vi "Data Acquisition.vi"() -> ()   [LabVIEW 2019]
uses:
  <vilib>/vision/Avi.llb/IMAQ AVI2 Refnum.ctl
  <vilib>/vision/Image Controls.llb/IMAQ Image.ctl
  <vilib>/Instr/_visa.llb/VISA Configure Serial Port (Instr).vi
panel:
  out "slowdata2":refnum<queue>
  out "slow frame":T1
  out "String":string="file:///C:\\Users\\ThymeLab\\Desktop\\omr_movies\\vdark50_vlight200_Rev.avi"
  in  "stop 2":bool
  in  "VLC Reference":refnum<k7>
  out "COMport":refnum<visa-resource-name>="COM4"
  out "hsframe":T1
  out "AVI Refnum":T2
  out "time log":refnum<file>
  out "slowdata":refnum<queue>
  out "integral1":refnum<queue>
  out "centroids1":refnum<queue>
  out "slowdisplay":refnum<queue>
  out "threshDisplay1":refnum<queue>
  in  "Tab Control":enum32{"Main View", "Files to load/save"}(tab)=enum."Files to load/save"
  out "Image":T1(plugin-control)
  in  "Ring":u16(ring) items=["Raw", "Diff Threshold", "Integrated Motion"]
  in  "stop":bool
  out "Buffers":i32(slide) scale=0.0..100.0
  out "Intensity Graph":u32[][](graph)
  out "movieindex":dbl
  in  "High Speed Movie Path":path=path "C:/Users/ThymeLab/Desktop/Box12/hsmovie"
  in  "ROI Refernce Image 1":path=path "C:/Users/ThymeLab/Desktop/Box12/Box12.png"
  in  "Load Experimental Parameters":path=path "C:/Users/ThymeLab/Desktop/Box12/fulltestrun_final_01_27_2020"
  in  "Load ROI Data":path=path "C:/Users/ThymeLab/Desktop/Box12/rois"
  in  "Log File Base Name":path=path "C:/Users/ThymeLab/Desktop/Box12/testlog"
  in  "diff threshold":dbl=3.0
  out "modhspath":path=path "C:/Users/ThymeLab/Desktop/Box1/hsmovieSun, Jun 14, 2020"
  in  "Teensy COM":refnum<visa-resource-name>="COM3"
  out "doQueue1":refnum<queue>
  out "hsdata":refnum<queue>
  in  "Folder containing stimulaton movies":path
  in  "Movie to Play":dbl
  in  "Pause":bool
  out "motion log":refnum<file>
  out "centroid log":refnum<file>
  out "ROIs":T3={[0, 0, 1088, 660], [{"Contour Type"=0, "ROI Type"=12, [32, 2, 115, 83, 90000]}, {"Contour Type"=0, "ROI Type"=12, [32, 83, 115, 164, 90000]}, {"Contour Type"=0, "ROI Type"=12, [32, 165, 115, 246, 90000]}, {"Contour Type"=0, "ROI Type"=12, [32, 246, 115, 327, 90000]}, {"Contour Type"=0, "ROI Type"=12, [32, 328, 116, 408, 90000]}, {"Contour Type"=0, "ROI Type"=12, [33, 409, 116, 490, 90000]}, {"Contour Type"=0, "ROI Type"=12, [33, 490, 116, 571, 90000]}, {"Contour Type"=0, "ROI Type"=12, [33, 572, 116, 653, 90000]}, {"Contour Type"=0, "ROI Type"=12, [116, 2, 199, 83, 90000]}, {"Contour Type"=0, "ROI Type"=12, [116, 83, 199, 164, 90000]}, {"Contour Type"=0, "ROI Type"=12, [116, 165, 199, 246, 90000]}, {"Contour Type"=0, "ROI Type"=12, [116, 246, 199, 327, 90000]}, {"Contour Type"=0, "ROI Type"=12, [116, 328, 199, 408, 90000]}, {"Contour Type"=0, "ROI Type"=12, [116, 409, 199, 490, 90000]}, {"Contour Type"=0, "ROI Type"=12, [116, 490, 199, 571, 90000]}, {"Contour Type"=0, "ROI Type"=12, [117, 572, 200, 653, 90000]}, {"Contour Type"=0, "ROI Type"=12, [199, 2, 282, 83, 90000]}, {"Contour Type"=0, "ROI Type"=12, [199, 83, 282, 164, 90000]}, {"Contour Type"=0, "ROI Type"=12, [200, 165, 283, 246, 90000]}, {"Contour Type"=0, "ROI Type"=12, [200, 246, 283, 327, 90000]}, {"Contour Type"=0, "ROI Type"=12, [200, 328, 283, 408, 90000]}, {"Contour Type"=0, "ROI Type"=12, [200, 409, 283, 490, 90000]}, {"Contour Type"=0, "ROI Type"=12, [200, 490, 283, 571, 90000]}, {"Contour Type"=0, "ROI Type"=12, [200, 572, 283, 653, 90000]}, {"Contour Type"=0, "ROI Type"=12, [283, 2, 366, 83, 90000]}, {"Contour Type"=0, "ROI Type"=12, [283, 83, 366, 164, 90000]}, {"Contour Type"=0, "ROI Type"=12, [283, 165, 366, 246, 90000]}, {"Contour Type"=0, "ROI Type"=12, [283, 246, 366, 327, 90000]}, {"Contour Type"=0, "ROI Type"=12, [284, 328, 366, 408, 90000]}, {"Contour Type"=0, "ROI Type"=12, [284, 409, 367, 490, 90000]}, {"Contour Type"=0, "ROI Type"=12, [284, 490, 367, 571, 90000]}, {"Contour Type"=0, "ROI Type"=12, [284, 572, 367, 653, 90000]}, {"Contour Type"=0, "ROI Type"=12, [367, 2, 450, 83, 90000]}, {"Contour Type"=0, "ROI Type"=12, [367, 83, 450, 164, 90000]}, {"Contour Type"=0, "ROI Type"=12, [367, 165, 450, 246, 90000]}, {"Contour Type"=0, "ROI Type"=12, [367, 246, 450, 327, 90000]}, {"Contour Type"=0, "ROI Type"=12, [367, 328, 450, 408, 90000]}, {"Contour Type"=0, "ROI Type"=12, [367, 409, 450, 490, 90000]}, {"Contour Type"=0, "ROI Type"=12, [367, 490, 450, 571, 90000]}, {"Contour Type"=0, "ROI Type"=12, [368, 572, 451, 653, 90000]}, {"Contour Type"=0, "ROI Type"=12, [450, 2, 533, 83, 90000]}, {"Contour Type"=0, "ROI Type"=12, [450, 83, 533, 164, 90000]}, {"Contour Type"=0, "ROI Type"=12, [451, 165, 534, 246, 90000]}, {"Contour Type"=0, "ROI Type"=12, [451, 246, 534, 327, 90000]}, {"Contour Type"=0, "ROI Type"=12, [451, 328, 534, 408, 90000]}, {"Contour Type"=0, "ROI Type"=12, [451, 409, 534, 490, 90000]}, {"Contour Type"=0, "ROI Type"=12, [451, 490, 534, 571, 90000]}, {"Contour Type"=0, "ROI Type"=12, [451, 572, 534, 653, 90000]}, {"Contour Type"=0, "ROI Type"=12, [534, 2, 617, 83, 90000]}, {"Contour Type"=0, "ROI Type"=12, [534, 83, 617, 164, 90000]}, {"Contour Type"=0, "ROI Type"=12, [534, 165, 617, 246, 90000]}, {"Contour Type"=0, "ROI Type"=12, [534, 246, 617, 327, 90000]}, {"Contour Type"=0, "ROI Type"=12, [534, 328, 618, 408, 90000]}, {"Contour Type"=0, "ROI Type"=12, [535, 409, 618, 490, 90000]}, {"Contour Type"=0, "ROI Type"=12, [535, 490, 618, 571, 90000]}, {"Contour Type"=0, "ROI Type"=12, [535, 572, 618, 653, 90000]}, {"Contour Type"=0, "ROI Type"=12, [618, 2, 701, 83, 90000]}, {"Contour Type"=0, "ROI Type"=12, [618, 83, 701, 164, 90000]}, {"Contour Type"=0, "ROI Type"=12, [618, 165, 701, 246, 90000]}, {"Contour Type"=0, "ROI Type"=12, [618, 246, 701, 327, 90000]}, {"Contour Type"=0, "ROI Type"=12, [618, 328, 701, 408, 90000]}, {"Contour Type"=0, "ROI Type"=12, [618, 409, 701, 490, 90000]}, {"Contour Type"=0, "ROI Type"=12, [618, 490, 701, 571, 90000]}, {"Contour Type"=0, "ROI Type"=12, [619, 572, 702, 653, 90000]}, {"Contour Type"=0, "ROI Type"=12, [701, 2, 784, 83, 90000]}, {"Contour Type"=0, "ROI Type"=12, [701, 83, 784, 164, 90000]}, {"Contour Type"=0, "ROI Type"=12, [702, 165, 785, 246, 90000]}, {"Contour Type"=0, "ROI Type"=12, [702, 246, 785, 327, 90000]}, {"Contour Type"=0, "ROI Type"=12, [702, 328, 785, 408, 90000]}, {"Contour Type"=0, "ROI Type"=12, [702, 409, 785, 490, 90000]}, {"Contour Type"=0, "ROI Type"=12, [702, 490, 785, 571, 90000]}, {"Contour Type"=0, "ROI Type"=12, [702, 572, 785, 653, 90000]}, {"Contour Type"=0, "ROI Type"=12, [785, 2, 868, 83, 90000]}, {"Contour Type"=0, "ROI Type"=12, [785, 83, 868, 164, 90000]}, {"Contour Type"=0, "ROI Type"=12, [785, 165, 868, 246, 90000]}, {"Contour Type"=0, "ROI Type"=12, [785, 246, 868, 327, 90000]}, {"Contour Type"=0, "ROI Type"=12, [786, 328, 868, 408, 90000]}, {"Contour Type"=0, "ROI Type"=12, [786, 409, 869, 490, 90000]}, {"Contour Type"=0, "ROI Type"=12, [786, 490, 869, 571, 90000]}, {"Contour Type"=0, "ROI Type"=12, [786, 572, 869, 653, 90000]}, {"Contour Type"=0, "ROI Type"=12, [869, 2, 952, 83, 90000]}, {"Contour Type"=0, "ROI Type"=12, [869, 83, 952, 164, 90000]}, {"Contour Type"=0, "ROI Type"=12, [869, 165, 952, 246, 90000]}, {"Contour Type"=0, "ROI Type"=12, [869, 246, 952, 327, 90000]}, {"Contour Type"=0, "ROI Type"=12, [869, 328, 952, 408, 90000]}, {"Contour Type"=0, "ROI Type"=12, [869, 409, 952, 490, 90000]}, {"Contour Type"=0, "ROI Type"=12, [869, 490, 952, 571, 90000]}, {"Contour Type"=0, "ROI Type"=12, [870, 572, 953, 653, 90000]}, {"Contour Type"=0, "ROI Type"=12, [952, 2, 1035, 83, 90000]}, {"Contour Type"=0, "ROI Type"=12, [952, 83, 1035, 164, 90000]}, {"Contour Type"=0, "ROI Type"=12, [953, 165, 1036, 246, 90000]}, {"Contour Type"=0, "ROI Type"=12, [953, 246, 1036, 327, 90000]}, {"Contour Type"=0, "ROI Type"=12, [953, 328, 1036, 408, 90000]}, {"Contour Type"=0, "ROI Type"=12, [953, 409, 1036, 490, 90000]}, {"Contour Type"=0, "ROI Type"=12, [953, 490, 1036, 571, 90000]}, {"Contour Type"=0, "ROI Type"=12, [953, 572, 1036, 653, 90000]}]}
  in  "roi data cluster":T3
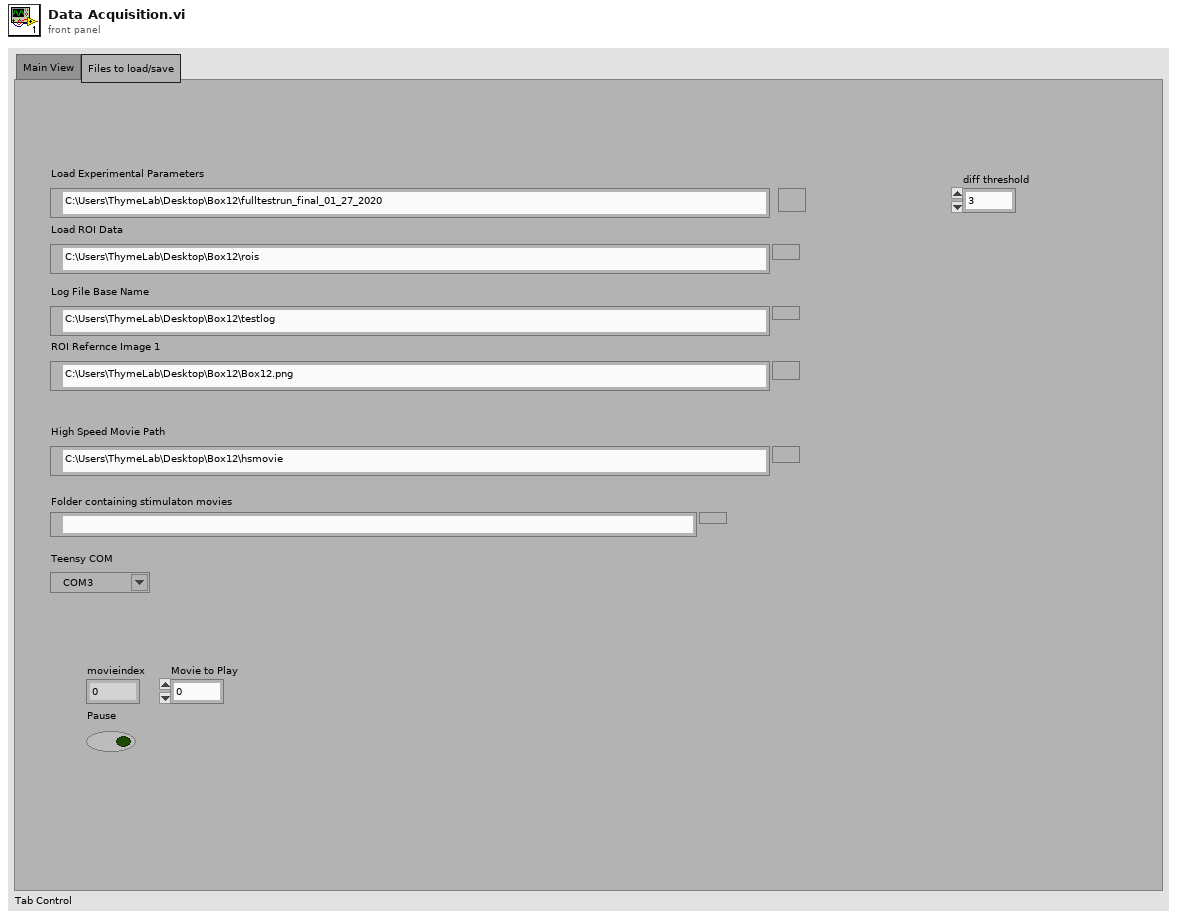
[diagram p1: front panel]
types:
  T1 = typedef "IMAQ Image.ctl" = refnum<image>
  T2 = typedef "IMAQ AVI2 Refnum.ctl" = refnum<k20>
  T3 = cluster{i32[], cluster{"Contour Type":u32, "ROI Type":u32, i32[]}[]}
  T4 = enum32{"Invalid", "Standard", "Closed", "Hidden", "Minimized", "Maximized"}
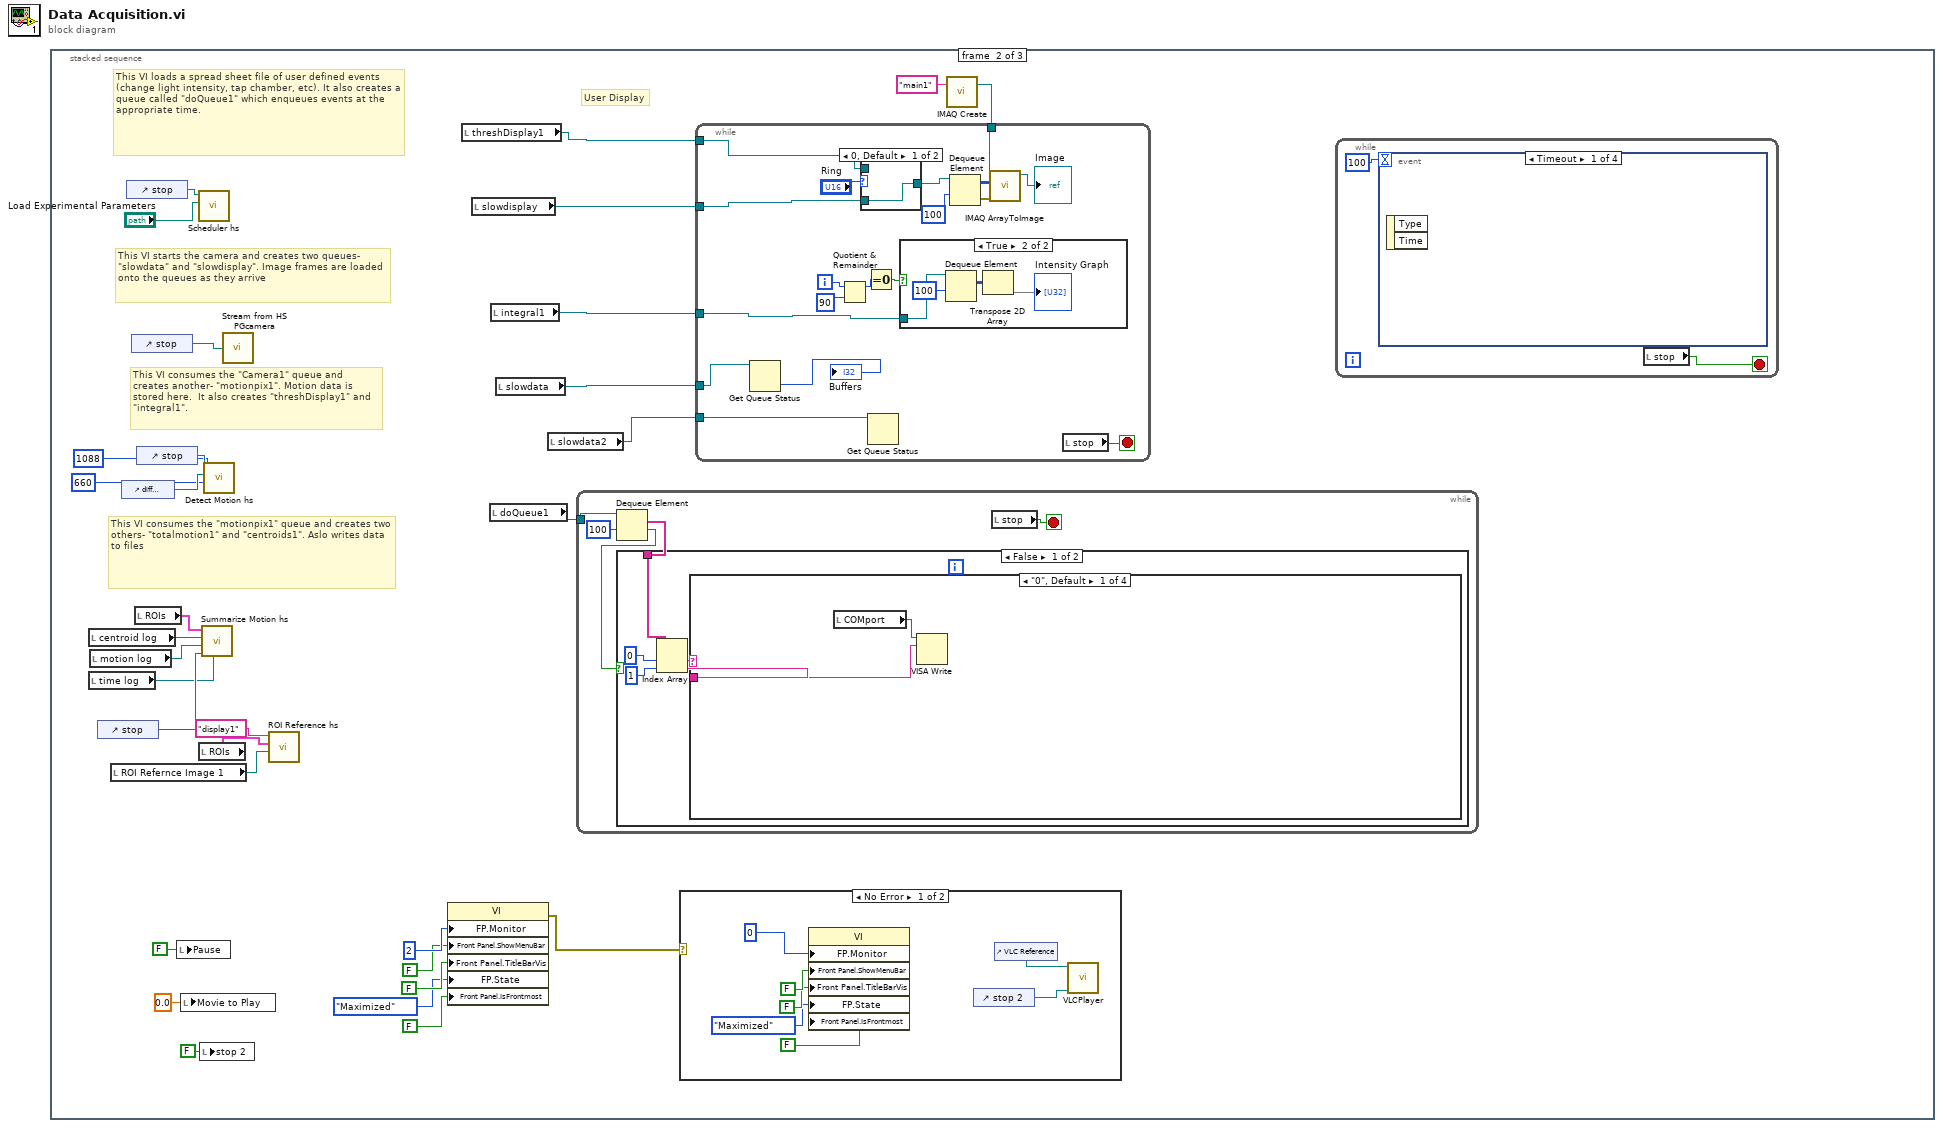
[diagram p0: block diagram]
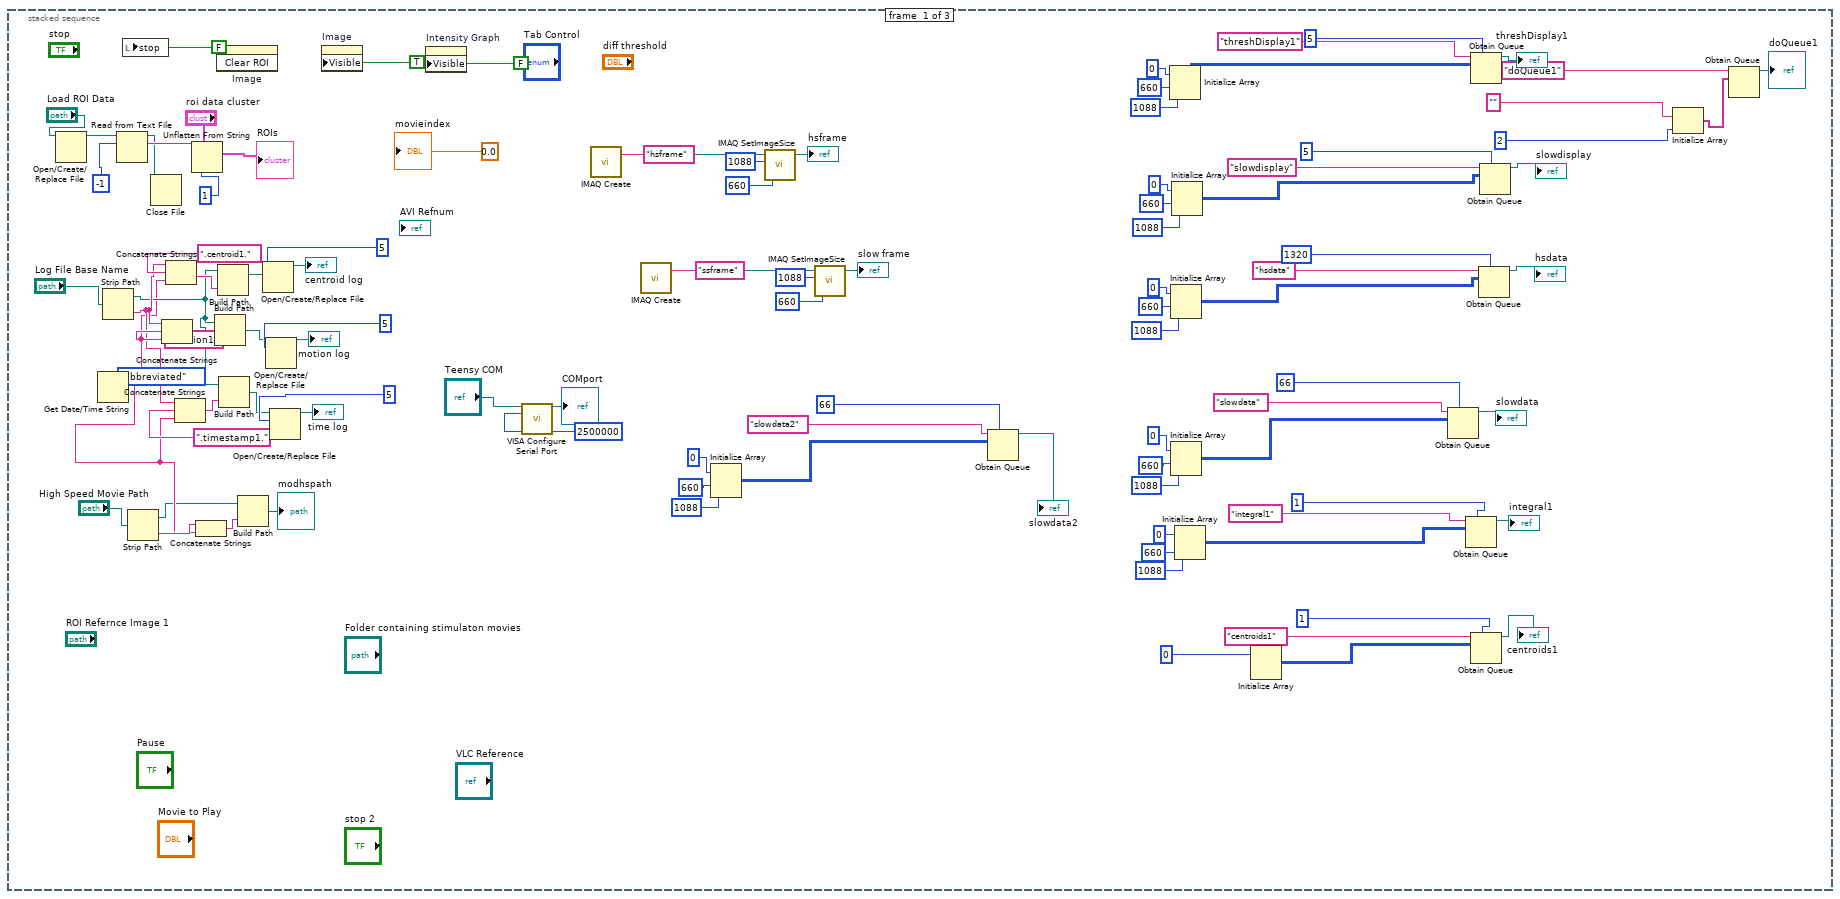
[diagram p2: hidden frame]
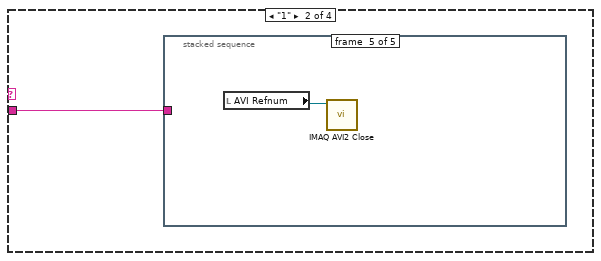
[diagram p4: hidden frame]
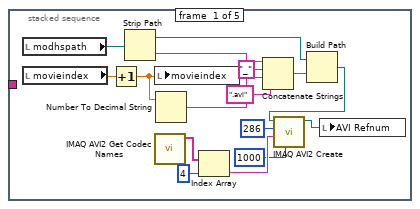
[diagram p5: hidden frame]
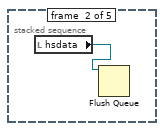
[diagram p6: hidden frame]
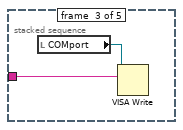
[diagram p7: hidden frame]
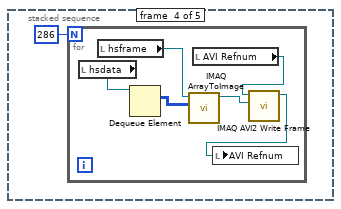
[diagram p8: hidden frame]
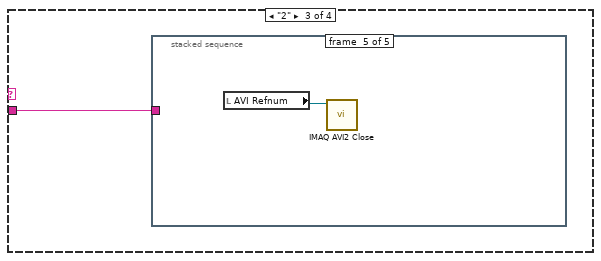
[diagram p9: hidden frame]
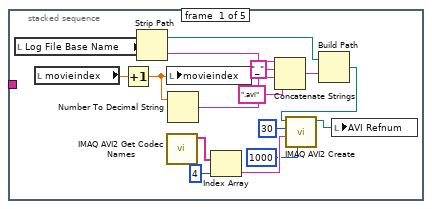
[diagram p10: hidden frame]
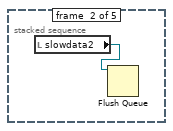
[diagram p11: hidden frame]
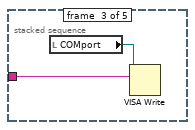
[diagram p12: hidden frame]
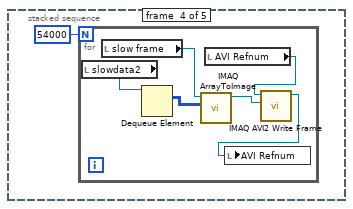
[diagram p13: hidden frame]
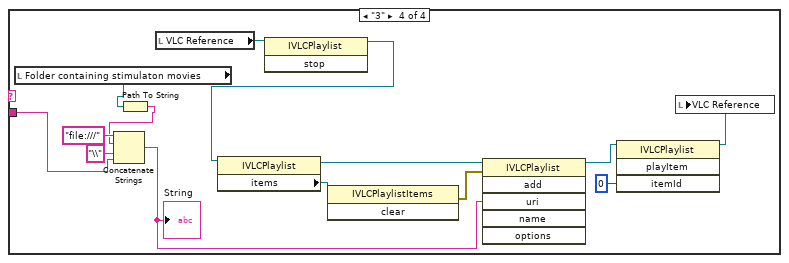
[diagram p14: hidden frame]
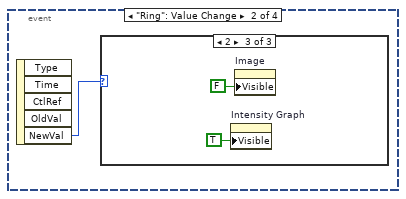
[diagram p16: hidden frame]
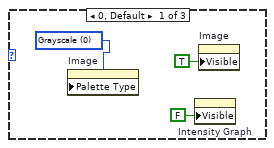
[diagram p17: hidden frame]
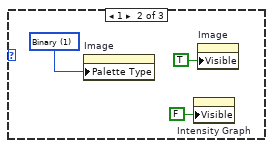
[diagram p18: hidden frame]
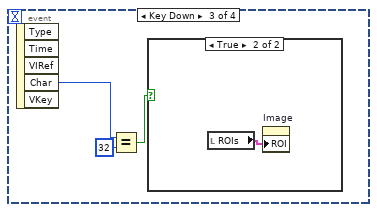
[diagram p19: hidden frame]
diagram:
  n1 = stacked-sequence {
    frame #0 {
      n2 = Open/Create/Replace File(file path (use dialog)="Load ROI Data") -> (refnum out=w97:refnum<file>)  [unwired: 5 in, 2 out]
      n3 = Get Date/Time String(date format (0)=enum16{"short", "long", "abbreviated"}."abbreviated") -> (date string=w31:string)  [unwired: 2 in, 1 out]
      n4 = Strip Path(path="Log File Base Name") -> (stripped path=w45:path, name=w47:string)
      n5 = Read from Text File(file (use dialog)=w97, count=-1) -> (refnum out=w99:refnum<file>, text=w100:string)  [unwired: 2 in, 2 out]
      n6 = local write "stop"(FALSE ("stop")) -> ()
      n7 = Strip Path(path="High Speed Movie Path") -> (stripped path=w29:path, name=w32:string)
      n8 = Close File(refnum=w99) -> ()  [unwired: 1 in, 2 out]
      n9 = Concatenate Strings(w47, ".motion1.", w31) -> (w88:string)
      n10 = Concatenate Strings(w47, ".centroid1.", w31) -> (w89:string)
      n11 = Concatenate Strings(w47, ".timestamp1." ("string"), w31) -> (w44:string)
      n12 = Unflatten From String(type="roi data cluster", binary string=w100, byte order (0:big-endian, network order)=1) -> (value=→"ROIs":T3)  [unwired: 2 in, 2 out]
      n13 = Concatenate Strings(w32, w31) -> (w30:string)
      n14 = Build Path(base path=w45, name or relative path=w88) -> (appended path=w84:path)
      n15 = invoke on="Image" class="ImageControl" method="Clear ROI"() -> ()  [unwired: 3 in, 3 out]
      n16 = Build Path(base path=w45, name or relative path=w89) -> (appended path=w87:path)
      n17 = Build Path(base path=w45, name or relative path=w44) -> (appended path=w42:path)
      n18 = Build Path(base path=w29, name or relative path=w30) -> (appended path=→"modhspath":path)
      n19 = Open/Create/Replace File(file path (use dialog)=w87, operation (0:open)=5 ("count")) -> (refnum out=→"centroid log":refnum<file>)  [unwired: 4 in, 2 out]
      n20 = Open/Create/Replace File(file path (use dialog)=w84, operation (0:open)=5 ("count")) -> (refnum out=→"motion log":refnum<file>)  [unwired: 4 in, 2 out]
      n21 = Open/Create/Replace File(file path (use dialog)=w42, operation (0:open)=5 ("count")) -> (refnum out=→"time log":refnum<file>)  [unwired: 4 in, 2 out]
      n22 = property on="Image" class="ImageControl"("Visible"=TRUE) -> ()  [unwired: 2 in, 2 out]
      n23 = property on="Intensity Graph" class="IntGraph (strict)"("Visible"=FALSE) -> ()  [unwired: 2 in, 2 out]
      n24 = call-poly "VISA Configure Serial Port"("VISA resource name"="Teensy COM", "baud rate (9600)"=u32 2500000) -> ("VISA resource name out"=→"COMport":refnum<visa-resource-name>)  [unwired: 12 in, 1 out]
      n25 = call "IMAQ Create"("Image Name"="hsframe") -> ("New Image"=w25:T1)  [unwired: 4 in, 1 out]
      n26 = call "IMAQ Create"("Image Name"="ssframe") -> ("New Image"=w11:T1)  [unwired: 4 in, 1 out]
      n27 = Initialize Array(i16 0 ("element"), 660 ("dimension size"), 1088 ("dimension size")) -> (w1:i16[][])
      n28 = call "IMAQ SetImageSize"("Y Resolution"=660, "X Resolution"=1088, "Image"=w25) -> ("Image Out"=→"hsframe":T1)  [unwired: 2 in, 1 out]
      n29 = call "IMAQ SetImageSize"("Y Resolution"=660, "X Resolution"=1088, "Image"=w11) -> ("Image Out"=→"slow frame":T1)  [unwired: 2 in, 1 out]
      n30 = Obtain Queue(max queue size (-1, unlimited)=66, name (unnamed)="slowdata2", element data type=w1) -> (queue out=→"slowdata2":refnum<queue>)  [unwired: 2 in, 2 out]
      n31 = Initialize Array(u8 0 ("element"), 660 ("dimension size"), 1088 ("dimension size")) -> (w75:u8[][])
      n32 = Initialize Array(u8 0 ("element"), 660 ("dimension size"), 1088 ("dimension size")) -> (w40:u8[][])
      n33 = Initialize Array(i16 0 ("element"), 660 ("dimension size"), 1088 ("dimension size")) -> (w48:i16[][])
      n34 = Initialize Array(u8 0 ("element"), 660 ("dimension size"), 1088 ("dimension size")) -> (w67:u8[][])
      n35 = Initialize Array(u32 0 ("element"), 660 ("dimension size"), 1088 ("dimension size")) -> (w61:u32[][])
      n36 = Initialize Array(u16 0 ("element")) -> (w49:u16[][])  [unwired: 2 in]
      n37 = Obtain Queue(max queue size (-1, unlimited)=66, name (unnamed)="slowdata", element data type=w48) -> (queue out=→"slowdata":refnum<queue>)  [unwired: 2 in, 2 out]
      n38 = Obtain Queue(max queue size (-1, unlimited)=1, name (unnamed)="integral1", element data type=w61) -> (queue out=→"integral1":refnum<queue>)  [unwired: 2 in, 2 out]
      n39 = Obtain Queue(max queue size (-1, unlimited)=5, name (unnamed)="threshDisplay1", element data type=w75) -> (queue out=→"threshDisplay1":refnum<queue>)  [unwired: 2 in, 2 out]
      n40 = Obtain Queue(max queue size (-1, unlimited)=1, name (unnamed)="centroids1", element data type=w49) -> (queue out=→"centroids1":refnum<queue>)  [unwired: 2 in, 2 out]
      n41 = Obtain Queue(max queue size (-1, unlimited)=1320, name (unnamed)="hsdata", element data type=w40) -> (queue out=→"hsdata":refnum<queue>)  [unwired: 2 in, 2 out]
      n42 = Obtain Queue(max queue size (-1, unlimited)=5, name (unnamed)="slowdisplay", element data type=w67) -> (queue out=→"slowdisplay":refnum<queue>)  [unwired: 2 in, 2 out]
      n43 = Initialize Array("", 2 ("dimension size")) -> (w16:string[])
      n44 = Obtain Queue(name (unnamed)="doQueue1", element data type=w16) -> (queue out=→"doQueue1":refnum<queue>)  [unwired: 3 in, 2 out]
      "movieindex" <- 0.0 ("movieindex")
    }
    frame #1 {
      # "User Display"
      # "This VI consumes the \"motionpix1\" queue and creates two others- \"totalmotion1\" and \"centroids1\". Aslo writes data to files"
      # "This VI consumes the \"Camera1\" queue and creates another- \"motionpix1\". Motion data is stored here.  It also creates \"threshDisplay1\" and \"integral1\"."
      # "This VI starts the camera and creates two queues- \"slowdata\" and \"slowdisplay\". Image frames are loaded onto the queues as they arrive"
      # "This VI loads a spread sheet file of user defined events (change light intensity, tap chamber, etc). It also creates a queue called \"doQueue1\" which enqueues events at the appropriate time."
      n45 = local read "centroid log"() -> (w127:refnum<file>)
      n46 = local read "time log"() -> (w116:refnum<file>)
      n47 = local read "motion log"() -> (w126:refnum<file>)
      n48 = control-ref of="stop"() -> (w125:refnum<vi>)
      n49 = local read "ROI Refernce Image 1"() -> (w119:path)
      n50 = control-ref of="diff threshold"() -> (w130:refnum<vi>)
      n51 = control-ref of="stop"() -> (w129:refnum<vi>)
      n52 = control-ref of="stop"() -> (w115:refnum<vi>)
      n53 = local read "ROIs"() -> (w128:T3)
      n54 = control-ref of="stop"() -> (w131:refnum<vi>)
      n55 = local write "Pause"(FALSE ("Pause")) -> ()
      n56 = local write "Movie to Play"(0.0 ("Movie to Play")) -> ()
      n57 = call "Scheduler hs.vi"("Load Experimental Parameters"="Load Experimental Parameters", "External Stop"=w129) -> ()  [unwired: 10 in]
      n58 = local read "ROIs"() -> (w118:T3)
      n59 = local write "stop 2"(FALSE ("stop")) -> ()
      n60 = call "Summarize Motion hs.vi"("time log"=w116, "external stop"=w125, "motion log"=w126, "centroid log"=w127, "roi data cluster"=w128) -> ()  [unwired: 7 in]
      n61 = call "Detect Motion hs.vi"("yres"=660, "xres"=1088, "thresh 1"=w130, "external stop"=w131) -> ()  [unwired: 8 in]
      n62 = call "Stream from HS PGcamera.vi"("External Stop"=w115) -> ()  [unwired: 3 in]
      n63 = call "ROI Reference hs.vi"("Path"=w119, "ROIs"=w118, "queue name"="display1") -> ()  [unwired: 8 in, 1 out]
      n64 = property class="VI"("FP.Monitor"=u16 2 ("Front Panel Window:Monitor"), "Front Panel.ShowMenuBar"=FALSE ("Front Panel Window:Show Menu Bar"), "Front Panel.TitleBarVis"=FALSE ("Front Panel Window:Title Bar Visible"), "FP.State"=T4."Maximized" ("Front Panel Window:State"), "Front Panel.IsFrontmost"=FALSE ("Front Panel Window:Is Frontmost")) -> (error out=w104:errorcluster)  [unwired: 2 in, 1 out]
      n65 = local read "threshDisplay1"() -> (w124:refnum<queue>)
      n66 = local read "slowdisplay"() -> (w123:refnum<queue>)
      n67 = local read "doQueue1"() -> (w120:refnum<queue>)
      n68 = local read "integral1"() -> (w122:refnum<queue>)
      n69 = local read "slowdata"() -> (w121:refnum<queue>)
      n70 = local read "slowdata2"() -> (w103:refnum<queue>)
      n71 = while {
        tunnel: w120 -> [w145]
        stop <- w146 stop-if-true
        n72 = Dequeue Element(queue=w145, timeout in ms (-1)=100) -> (element=w143:string[], timed out?=w142:bool)  [unwired: 1 in, 2 out]
        n73 = case shown="False" w142 {
          tunnel: w143 -> [w151 _]
          frame False {
            n74 = Index Array(array=w151, index #1=0 ("index"), index #2=1 ("index")) -> (element #1=w148:string, element #2=w147:string)
            n75 = case shown="\"0\", Default" w148 {
              tunnel: w147 -> [w152 w154 w182 w211]
              frame "0", Default {
                n76 = local read "COMport"() -> (w153:refnum<visa-resource-name>)
                n77 = VISA Write(VISA resource name=w153, write buffer=w152) -> ()  [unwired: 1 in, 3 out]
              }
              frame "1" {
                n78 = stacked-sequence {
                  tunnel: w154 -> [_ _ w173 _ _]
                  frame #0 {
                    n79 = local read "modhspath"() -> (w169:path)
                    n80 = local read "movieindex"() -> (w170:dbl)
                    n81 = Increment(x=w170) -> (x+1=w168:dbl)
                    n82 = Strip Path(path=w169) -> (stripped path=w162:path, name=w167:string)
                    n83 = local write "movieindex"(w168) -> ()
                    n84 = call "IMAQ AVI2 Get Codec Names"() -> ("Codec Names"=w159:string[])  [unwired: 10 in, 1 out]
                    n85 = Number To Decimal String(number=w168) -> (decimal integer string=w166:string)  [unwired: 1 in]
                    n86 = Index Array(array=w159, index=4) -> (element=w157:string)
                    n87 = Concatenate Strings(w167, "_" ("string"), w166, ".avi" ("string")) -> (w163:string)
                    n88 = Build Path(base path=w162, name or relative path=w163) -> (appended path=w161:path)
                    n89 = call "IMAQ AVI2 Create"("Quality"=1000, "Codec"=w157, "Frames Per Second"=u32 286, "AVI Path"=w161) -> ("AVI Refnum"=w155:T2)  [unwired: 6 in, 1 out]
                    n90 = local write "AVI Refnum"(w155) -> ()
                  }
                  frame #1 {
                    n91 = local read "hsdata"() -> (w171:refnum<queue>)
                    n92 = Flush Queue(queue=w171) -> ()  [unwired: 1 in, 3 out]
                  }
                  frame #2 {
                    n93 = local read "COMport"() -> (w172:refnum<visa-resource-name>)
                    n94 = VISA Write(VISA resource name=w172, write buffer=w173) -> ()  [unwired: 1 in, 3 out]
                  }
                  frame #3 {
                    n95 = for {
                      N: 286 -> [_]
                      n96 = local read "hsdata"() -> (w180:refnum<queue>)
                      n97 = local read "hsframe"() -> (w178:T1)
                      n98 = Dequeue Element(queue=w180) -> (element=w179:u8[][])  [unwired: 2 in, 3 out]
                      n99 = call "IMAQ ArrayToImage"("Image Pixels (U8)"=w179, "Image"=w178) -> ("Image Out"=w176:T1)  [unwired: 8 in, 1 out]
                      n100 = local read "AVI Refnum"() -> (w177:T2)
                      n101 = call "IMAQ AVI2 Write Frame"("Image"=w176, "AVI Refnum"=w177) -> ("AVI Refnum (duplicate)"=w175:T2)  [unwired: 7 in, 2 out]
                      n102 = local write "AVI Refnum"(w175) -> ()
                    }
                  }
                  frame #4 {
                    n103 = local read "AVI Refnum"() -> (w181:T2)
                    n104 = call "IMAQ AVI2 Close"("AVI Refnum"=w181) -> ()  [unwired: 10 in, 1 out]
                  }
                }
              }
              frame "2" {
                n105 = stacked-sequence {
                  tunnel: w182 -> [_ _ w201 _ _]
                  frame #0 {
                    n106 = local read "Log File Base Name"() -> (w197:path)
                    n107 = local read "movieindex"() -> (w198:dbl)
                    n108 = Increment(x=w198) -> (x+1=w196:dbl)
                    n109 = Strip Path(path=w197) -> (stripped path=w190:path, name=w195:string)
                    n110 = local write "movieindex"(w196) -> ()
                    n111 = call "IMAQ AVI2 Get Codec Names"() -> ("Codec Names"=w187:string[])  [unwired: 10 in, 1 out]
                    n112 = Number To Decimal String(number=w196) -> (decimal integer string=w194:string)  [unwired: 1 in]
                    n113 = Index Array(array=w187, index=4) -> (element=w185:string)
                    n114 = Concatenate Strings(w195, "_" ("string"), w194, ".avi" ("string")) -> (w191:string)
                    n115 = Build Path(base path=w190, name or relative path=w191) -> (appended path=w189:path)
                    n116 = call "IMAQ AVI2 Create"("Quality"=1000, "Codec"=w185, "Frames Per Second"=u32 30, "AVI Path"=w189) -> ("AVI Refnum"=w183:T2)  [unwired: 6 in, 1 out]
                    n117 = local write "AVI Refnum"(w183) -> ()
                  }
                  frame #1 {
                    n118 = local read "slowdata2"() -> (w199:refnum<queue>)
                    n119 = Flush Queue(queue=w199) -> ()  [unwired: 1 in, 3 out]
                  }
                  frame #2 {
                    n120 = local read "COMport"() -> (w200:refnum<visa-resource-name>)
                    n121 = VISA Write(VISA resource name=w200, write buffer=w201) -> ()  [unwired: 1 in, 3 out]
                  }
                  frame #3 {
                    n122 = for {
                      N: 54000 -> [_]
                      n123 = local read "slowdata2"() -> (w208:refnum<queue>)
                      n124 = local read "slow frame"() -> (w206:T1)
                      n125 = Dequeue Element(queue=w208) -> (element=w207:i16[][])  [unwired: 2 in, 3 out]
                      n126 = call "IMAQ ArrayToImage"("Image Pixels (U8)"=w207, "Image"=w206) -> ("Image Out"=w204:T1)  [unwired: 8 in, 1 out]
                      n127 = local read "AVI Refnum"() -> (w205:T2)
                      n128 = call "IMAQ AVI2 Write Frame"("Image"=w204, "AVI Refnum"=w205) -> ("AVI Refnum (duplicate)"=w203:T2)  [unwired: 7 in, 2 out]
                      n129 = local write "AVI Refnum"(w203) -> ()
                    }
                  }
                  frame #4 {
                    n130 = local read "AVI Refnum"() -> (w209:T2)
                    n131 = call "IMAQ AVI2 Close"("AVI Refnum"=w209) -> ()  [unwired: 10 in, 1 out]
                  }
                }
              }
              frame "3" {
                n132 = local read "Folder containing stimulaton movies"() -> (w215:path)
                n133 = Path To String(path=w215) -> (string=w213:string)
                n134 = Concatenate Strings("file:///" ("string"), w213, "\\" ("string"), w211) -> (w210:string)
                "String" <- w210
                n135 = local read "VLC Reference"() -> (w223:refnum<k7>)
                n136 = invoke class="IVLCPlaylist" method="stop"(reference=w223) -> (reference out=w222:refnum<k7>)  [unwired: 2 in, 2 out]
                n137 = property class="IVLCPlaylist"(reference=w222) -> (reference out=w219:refnum<k7>, "items"=w221:refnum<k7>)  [unwired: 1 in, 1 out]
                n138 = invoke class="IVLCPlaylistItems" method="clear"(reference=w221) -> (error out=w220:errorcluster)  [unwired: 2 in, 2 out]
                n139 = invoke class="IVLCPlaylist" method="add"(reference=w219, error in=w220, "uri"=w210) -> (reference out=w218:refnum<k7>)  [unwired: 3 in, 5 out]
                n140 = invoke class="IVLCPlaylist" method="playItem"(reference=w218, "itemId"=0) -> (reference out=w216:refnum<k7>)  [unwired: 2 in, 3 out]
                n141 = local write "VLC Reference"(w216) -> ()
              }
            }
          }
          frame True {
          }
        }
        n142 = local read "stop"() -> (w146:bool)
      }
      n143 = case shown="No Error" w104 {
        frame No Error {
          n144 = property class="VI"("FP.Monitor"=u16 0 ("Front Panel Window:Monitor"), "Front Panel.ShowMenuBar"=FALSE ("Front Panel Window:Show Menu Bar"), "Front Panel.TitleBarVis"=FALSE ("Front Panel Window:Title Bar Visible"), "FP.State"=T4."Maximized" ("Front Panel Window:State"), "Front Panel.IsFrontmost"=FALSE ("Front Panel Window:Is Frontmost")) -> ()  [unwired: 2 in, 2 out]
          n145 = control-ref of="stop 2"() -> (w140:refnum<vi>)
          n146 = control-ref of="VLC Reference"() -> (w141:refnum<vi>)
          n147 = call "VLCPlayer.vi"("stop ref in"=w140, "VLC Reference In"=w141) -> ()  [unwired: 10 in]
        }
        frame Error {
        }
      }
      n148 = call "IMAQ Create"("Image Name"="main1") -> ("New Image"=w132:T1)  [unwired: 4 in, 1 out]
      n149 = while {
        tunnel: w123 -> [w245]
        tunnel: w132 -> [w256]
        tunnel: w124 -> [w246]
        tunnel: w122 -> [w244]
        tunnel: w121 -> [w242]
        tunnel: w103 -> [w240]
        i -> [w241]
        stop <- w255 stop-if-true
        n150 = Get Queue Status(queue=w242) -> (# elements in queue=→"Buffers":i32)  [unwired: 2 in, 7 out]
        n151 = Quotient & Remainder(x=w241, y=90) -> (x-y*floor(x/y)=w248:i32)  [unwired: 1 out]
        n152 = case shown="0, Default" "Ring" {
          tunnel: w245 -> [w261 _]
          tunnel: [w261 w262] -> w251
          tunnel: w246 -> [_ w262]
          frame 0, Default {
          }
          frame 1 {
          }
        }
        n153 = Equal To 0?(x=w248) -> (x = 0?=w247:bool)
        n154 = Get Queue Status(queue=w240) -> ()  [unwired: 2 in, 8 out]
        n155 = case shown="True" w247 {
          tunnel: w244 -> [_ w260]
          frame False {
          }
          frame True {
            n156 = Dequeue Element(queue=w260, timeout in ms (-1)=100) -> (element=w258:u32[][])  [unwired: 1 in, 3 out]
            n157 = Transpose 2D Array(2D array=w258) -> (transposed array=→"Intensity Graph":u32[][])
          }
        }
        n158 = Dequeue Element(queue=w251, timeout in ms (-1)=100) -> (element=w252:u8[][], error out=w254:errorcluster)  [unwired: 1 in, 2 out]
        n159 = call "IMAQ ArrayToImage"("error in (no error)"=w254, "Image Pixels (U8)"=w252, "Image"=w256) -> ("Image Out"=→"Image":T1)  [unwired: 7 in, 1 out]
        n160 = local read "stop"() -> (w255:bool)
      }
      n161 = while {
        stop <- w225 stop-if-true
        n162 = event shown="[0] Timeout" {
          selector: _ -> [_ _ _ _]
          dyn-events: _ -> [_ _ _ _]
          timeout: 100 -> [_ _ _ _]
          event Timeout {
            n163 = event-data() -> ()  [unwired: 1 in, 2 out]
          }
          event "Ring": Value Change {
            n164 = event-data() -> ("NewVal"=w226:u16)  [unwired: 1 in, 4 out]
            n165 = case shown="2" w226 {
              frame 0, Default {
                w229 = u32 0 items=["Grayscale", "Binary", "Gradient", "Rainbow", "Temperature", "User Defined"] ("Palette:Palette Type")
                n166 = property on="Image" class="ImageControl"("Palette Type"=w229) -> ()  [unwired: 2 in, 2 out]
                n167 = property on="Intensity Graph" class="IntGraph (strict)"("Visible"=FALSE) -> ()  [unwired: 2 in, 2 out]
                n168 = property on="Image" class="ImageControl"("Visible"=TRUE) -> ()  [unwired: 2 in, 2 out]
              }
              frame 1 {
                w232 = u32 1 items=["Grayscale", "Binary", "Gradient", "Rainbow", "Temperature", "User Defined"] ("Palette:Palette Type")
                n169 = property on="Image" class="ImageControl"("Palette Type"=w232) -> ()  [unwired: 2 in, 2 out]
                n170 = property on="Intensity Graph" class="IntGraph (strict)"("Visible"=FALSE) -> ()  [unwired: 2 in, 2 out]
                n171 = property on="Image" class="ImageControl"("Visible"=TRUE) -> ()  [unwired: 2 in, 2 out]
              }
              frame 2 {
                n172 = property on="Intensity Graph" class="IntGraph (strict)"("Visible"=TRUE) -> ()  [unwired: 2 in, 2 out]
                n173 = property on="Image" class="ImageControl"("Visible"=FALSE) -> ()  [unwired: 2 in, 2 out]
              }
            }
          }
          event Key Down {
            n174 = event-data() -> ("Char"=w237:i16)  [unwired: 1 in, 4 out]
            n175 = Equal?(x=w237, y=i16 32) -> (x = y?=w235:bool)
            n176 = case shown="True" w235 {
              frame False {
              }
              frame True {
                n177 = local read "ROIs"() -> (w238:T3)
                n178 = property on="Image" class="ImageControl"("ROI"=w238) -> ()  [unwired: 2 in, 2 out]
              }
            }
          }
          event Key Up {
            n179 = event-data() -> ()  [unwired: 1 in, 7 out]
            n180 = invoke on="Image" class="ImageControl" method="Clear ROI"() -> ()  [unwired: 3 in, 3 out]
          }
        }
        n181 = local read "stop"() -> (w225:bool)
      }
    }
    frame #2 {
      n182 = local read "COMport"() -> (w263:refnum<visa-resource-name>)
      n183 = VISA Close(VISA resource name=w263) -> ()  [unwired: 1 in, 1 out]
    }
  }
